vi "RegisterDataSetsRoutedMessage_Send.vi"(7 "data event creator process name":string="CmsDataEventCreator", 8 "error in (no error)":errorcluster, 10 "RegisterDataSet":T1, 11 "Qbus in":refnum<class "Qbus.lvclass">) -> (0 "error out":errorcluster, 3 "Qbus out":refnum<class "Qbus.lvclass">)   [LabVIEW 2017, in "DataEventCreator.lvlib"]
doc: "Provides the TDMS Creator process with information about trends calculated from channel data. Trends must be registered with TDMS Creator, otherwise the TDMS Creator process does not write their values to file."
uses:
  <vilib>/addons/InsightCM/Devices/Shared/Common/DataEventCreator/DataEventCreator.lvlib
  <vilib>/addons/Qbus/Qbus.lvclass
  <vilib>/addons/InsightCM/Devices/Shared/Common/DataEventCreator/controls/RegisterDataSets.ctl
  <vilib>/addons/InsightCM/Devices/Shared/Cms/CmsDataEventCreator/controls/DataSetRegistry.ctl
  <vilib>/addons/InsightCM/Devices/Shared/Common/DataEvent/controls/DataSetType.ctl
  <vilib>/addons/InsightCM/Devices/Shared/Common/DataEvent/DataEvent.lvlib
  <vilib>/addons/InsightCM/Devices/Shared/Cms/CmsDataEventCreator/CmsDataEventCreator.lvlib
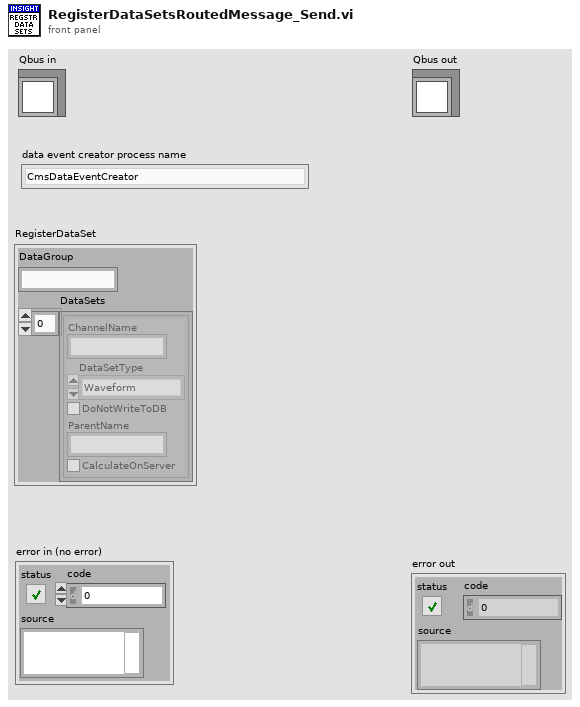
[diagram p1: front panel]
types:
  T1 = typedef "DataEventCreator.lvlib/RegisterDataSets.ctl" = cluster{"DataGroup":string, "DataSets":T2[]}
  T2 = typedef "CmsDataEventCreator.lvlib/DataSetRegistry.ctl" = cluster{"ChannelName":string, "DataSetType":T3, "DoNotWriteToDB":bool, "ParentName":string, "CalculateOnServer":bool}
  T3 = typedef "DataEvent.lvlib/DataSetType.ctl" = enum16{"Waveform", "SpeedProfile", "ThermalImage", "EmsaSweep"}
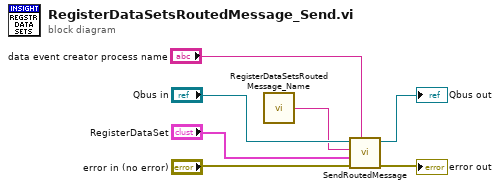
[diagram p0: block diagram]
diagram:
  n1 = call <vilib>:"RegisterDataSetsRoutedMessage_Name.vi"() -> ("message name"=w2:string)  [unwired: 5 in]
  n2 = call <vilib>:"SendRoutedMessage.vi"("listener process"="data event creator process name", "error in (no error)"="error in (no error)", "message value"="RegisterDataSet", "message name"=w2, "Qbus in"="Qbus in") -> ("error in (no error)"=→"error out":errorcluster, "Qbus out"=→"Qbus out":refnum<class "Qbus.lvclass">)  [unwired: 5 in]
